vi "String to U8.vi"(8 "error in":errorcluster, 11 "String":string) -> (0 "error out":errorcluster, 3 "U8":u8)   [LabVIEW 2024, in "Electronic Datasheet.lvlib"]
doc: "A string that contains the number to convert."
uses:
  Electronic Datasheet.lvlib
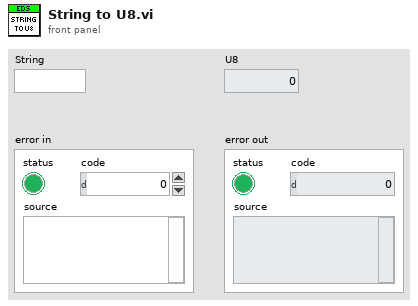
[diagram p1: front panel]
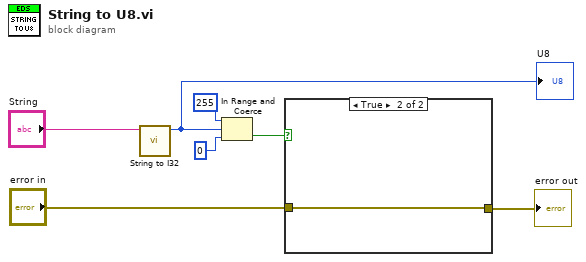
[diagram p0: block diagram]
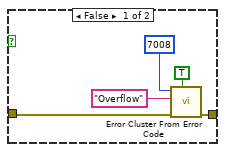
[diagram p2: hidden frame]
diagram:
  n1 = call "String to I32.vi"("String"="String") -> ("I32"=w3:i32)  [unwired: 10 in]
  "U8" <- w3
  n2 = In Range and Coerce(upper limit=255, x=w3, lower limit=0) -> (In Range?=w4:bool)  [unwired: 1 out]
  n3 = case shown="True" w4 {
    tunnel: "error in" -> [w12 w13]
    tunnel: [w8 w13] -> w1
    frame False {
      n4 = call <vilib>:"Error Cluster From Error Code.vi"("show call chain? (False)"=TRUE, "error in (no error)"=w12, "error message (\"\")"="Overflow" ("error message (\"\")"), "error code (0)"=7008) -> ("error out"=w8:errorcluster)  [unwired: 5 in]
    }
    frame True {
    }
  }
  "error out" <- w1
